vi "set_proxy.vi"(5 "username":string, 7 "password":string, 8 "error in":errorcluster, 9 "port":u16=8080, 10 "server":string, 11 "ClientBuilder in":refnum<class "ClientBuilder.lvclass">) -> (0 "error out":errorcluster, 2 "success":bool, 3 "ClientBuilder out":refnum<class "ClientBuilder.lvclass">)   [LabVIEW 2020, in "reqwest.lvlib" / "ClientBuilder.lvclass"]
uses:
  ClientBuilder.lvclass
  ClientBuilder.lvclass/ClientBuilder.ctl
  lv_reqwest_32.dll
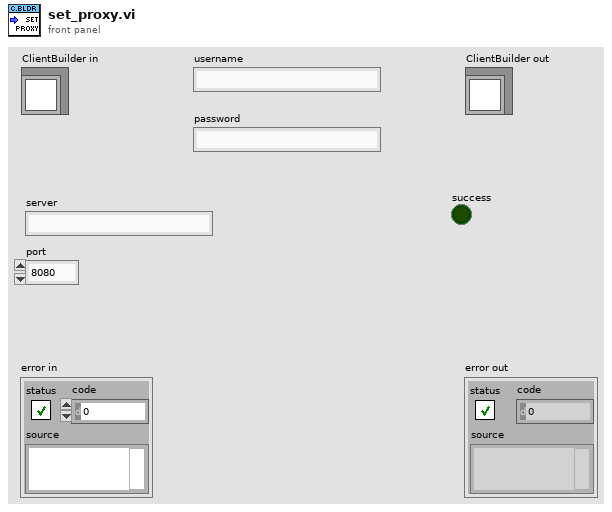
[diagram p1: front panel]
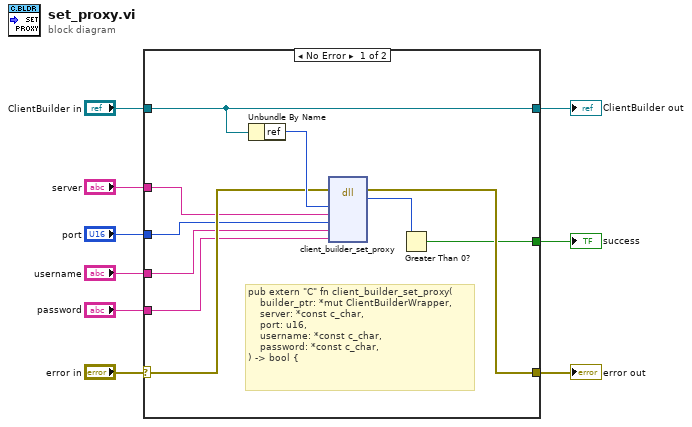
[diagram p0: block diagram]
diagram:
  n1 = case shown="No Error" "error in" {
    selector: "error in" -> [w16 w20]
    tunnel: "ClientBuilder in" -> [w17 w21]
    tunnel: [w19 w20] -> w6
    tunnel: [w17 w21] -> w7
    tunnel: [w14 _] -> w5
    tunnel: "server" -> [w13 _]
    tunnel: "port" -> [w12 _]
    tunnel: "username" -> [w11 _]
    tunnel: "password" -> [w10 _]
    frame No Error {
      # "pub extern \"C\" fn client_builder_set_proxy(\n    builder_ptr: *mut ClientBuilderWrapper,\n    server: *const c_char,\n    port: u16,\n    username: *const c_char,\n    password: *const c_char,\n) -> bool {"
      n2 = Unbundle By Name(w17) -> ("ref"=w18:u64)
      n3 = dll-call lib="C:/Projects/reqwest-rs-labview/lv_src/lv_reqwest_*.*" fn="client_builder_set_proxy"(error in=w16, "client_builder_ref"=w18, "server"=w13, "port"=w12, "username"=w11, "password"=w10) -> (error out=w19:errorcluster, "success"=w15:u8)  [unwired: 7 in, 1 out]
      n4 = Greater Than 0?(x=w15) -> (x > 0?=w14:bool)
    }
    frame Error {
    }
  }
  "error out" <- w6
  "ClientBuilder out" <- w7
  "success" <- w5
